vi "Reading_Temperature_Generatng_PWM.vi"() -> ()   [LabVIEW 2024]
uses:
  <vilib>/Instr/_visa.llb/VISA Configure Serial Port (Instr).vi
  <vilib>/regexp/Match Regular Expression.xnode
panel:
  out "Trepassing Temperature Alert":bool
  in  "Teperature Reference":dbl
  out "Temperature (*C)":dbl
  out "Humidity (%)":dbl
  in  "stop":bool
  in  "baud rate (9600)":u32=9600
  in  "COM Port":refnum<visa-resource-name>
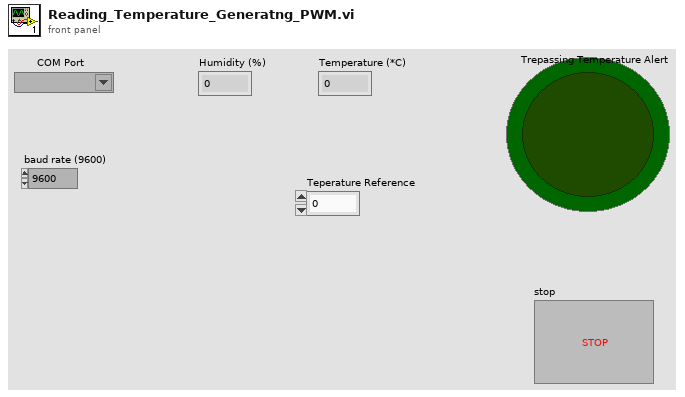
[diagram p1: front panel]
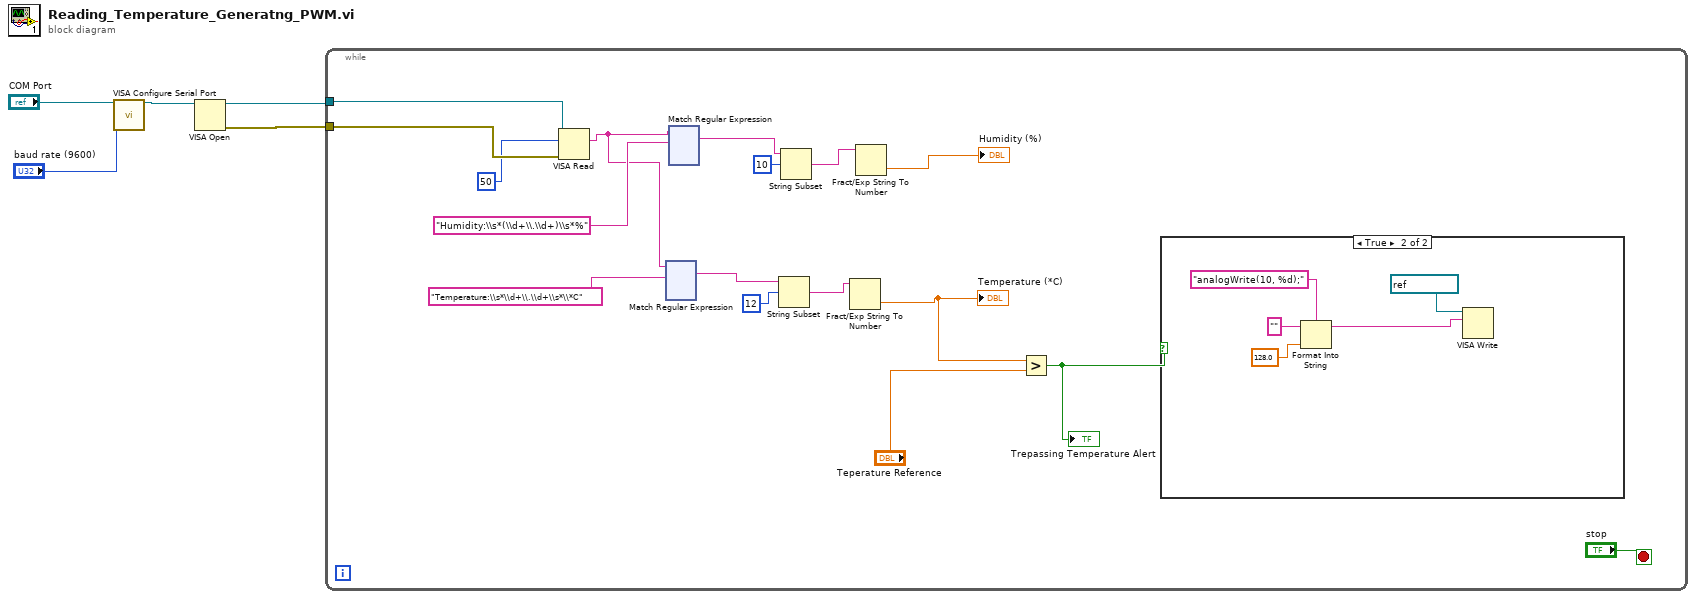
[diagram p0: block diagram]
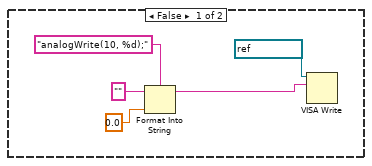
[diagram p2: hidden frame]
diagram:
  n1 = call-poly "VISA Configure Serial Port"("VISA resource name"="COM Port", "baud rate (9600)"="baud rate (9600)") -> ("VISA resource name out"=w4:refnum<visa-resource-name>)  [unwired: 12 in, 1 out]
  n2 = VISA Open(VISA resource name=w4) -> (VISA resource name=w3:refnum<visa-resource-name>, error out=w1:errorcluster)  [unwired: 4 in]
  n3 = while {
    tunnel: w3 -> [w7]
    tunnel: w1 -> [w22]
    stop <- "stop" stop-if-true
    n4 = VISA Read(VISA resource name=w7, byte count=u32 50, error in (no error)=w22) -> (read buffer=w14:string)  [unwired: 3 out]
    n5 = xnode "Match Regular Expression"("input string"=w14, "regular expression"="Temperature:\\s*\\d+\\.\\d+\\s*\\*C") -> ("whole match"=w12:string)  [unwired: 4 in, 4 out]
    n6 = xnode "Match Regular Expression"("input string"=w14, "regular expression"="Humidity:\\s*(\\d+\\.\\d+)\\s*%") -> ("whole match"=w17:string)  [unwired: 4 in, 4 out]
    n7 = String Subset(string=w12, offset (0)=12) -> (substring=w10:string)  [unwired: 1 in]
    n8 = String Subset(string=w17, offset (0)=10) -> (substring=w16:string)  [unwired: 1 in]
    n9 = Fract/Exp String To Number(string=w10) -> (number=w9:dbl)  [unwired: 3 in, 1 out]
    "Temperature (*C)" <- w9
    n10 = Fract/Exp String To Number(string=w16) -> (number=→"Humidity (%)":dbl)  [unwired: 3 in, 1 out]
    n11 = Greater?(x=w9, y="Teperature Reference") -> (0:w6:bool)
    "Trepassing Temperature Alert" <- w6
    n12 = case shown="True" w6 {
      frame False {
        n13 = Format Into String(format string="analogWrite(10, %d);", initial string="", 0.0 ("input 1")) -> (resulting string=w27:string)  [unwired: 1 in, 1 out]
        n14 = VISA Write(VISA resource name=refnum<visa-resource-name> "COM11", write buffer=w27) -> ()  [unwired: 1 in, 3 out]
      }
      frame True {
        n15 = Format Into String(format string="analogWrite(10, %d);", initial string="", 128.0 ("input 1")) -> (resulting string=w29:string)  [unwired: 1 in, 1 out]
        n16 = VISA Write(VISA resource name=refnum<visa-resource-name> "COM11", write buffer=w29) -> ()  [unwired: 1 in, 3 out]
      }
    }
  }
